vi "get scan info.vi"(5 "piezo z value":i16, 6 "tracking?":bool, 7 "counting photons?":bool, 8 "kalman to host":cluster{"kalman state":T1, "kalman update":bool}, 9 "current location":T3, 10 "scan specification":T2={"z resolution (pixels)"=1000, "iterations per pixel"=28, "iterations per z-scan (=zres*iterperpixel)"=50, "x resolution (pixels)"=100, "y resolution (pixels)"=80, "number of z-lines per volume"=30, "number of repetitions (volumes)"=5, "Pockels cell voltage (bits)"=-1, "Vx center (bits)"=0, "Vy center (bits)"=0, "Vx amplitude (bits)"=40, "Vy amplitude (bits)"=0, "lines to delay between scan start and output"=1, "LSB has acquire control"=FALSE, "Pockels cell bleach voltage"=0}, 11 "counter cluster":T5) -> (3 "scan info":T4)   [LabVIEW 2010]
uses:
  counter_cluster_tagResonant.ctl
  scan_command.ctl
  scan_specification_tagResonant.ctl
  FPGA tracking/integrating single axis kalman state.ctl
  scan message.ctl
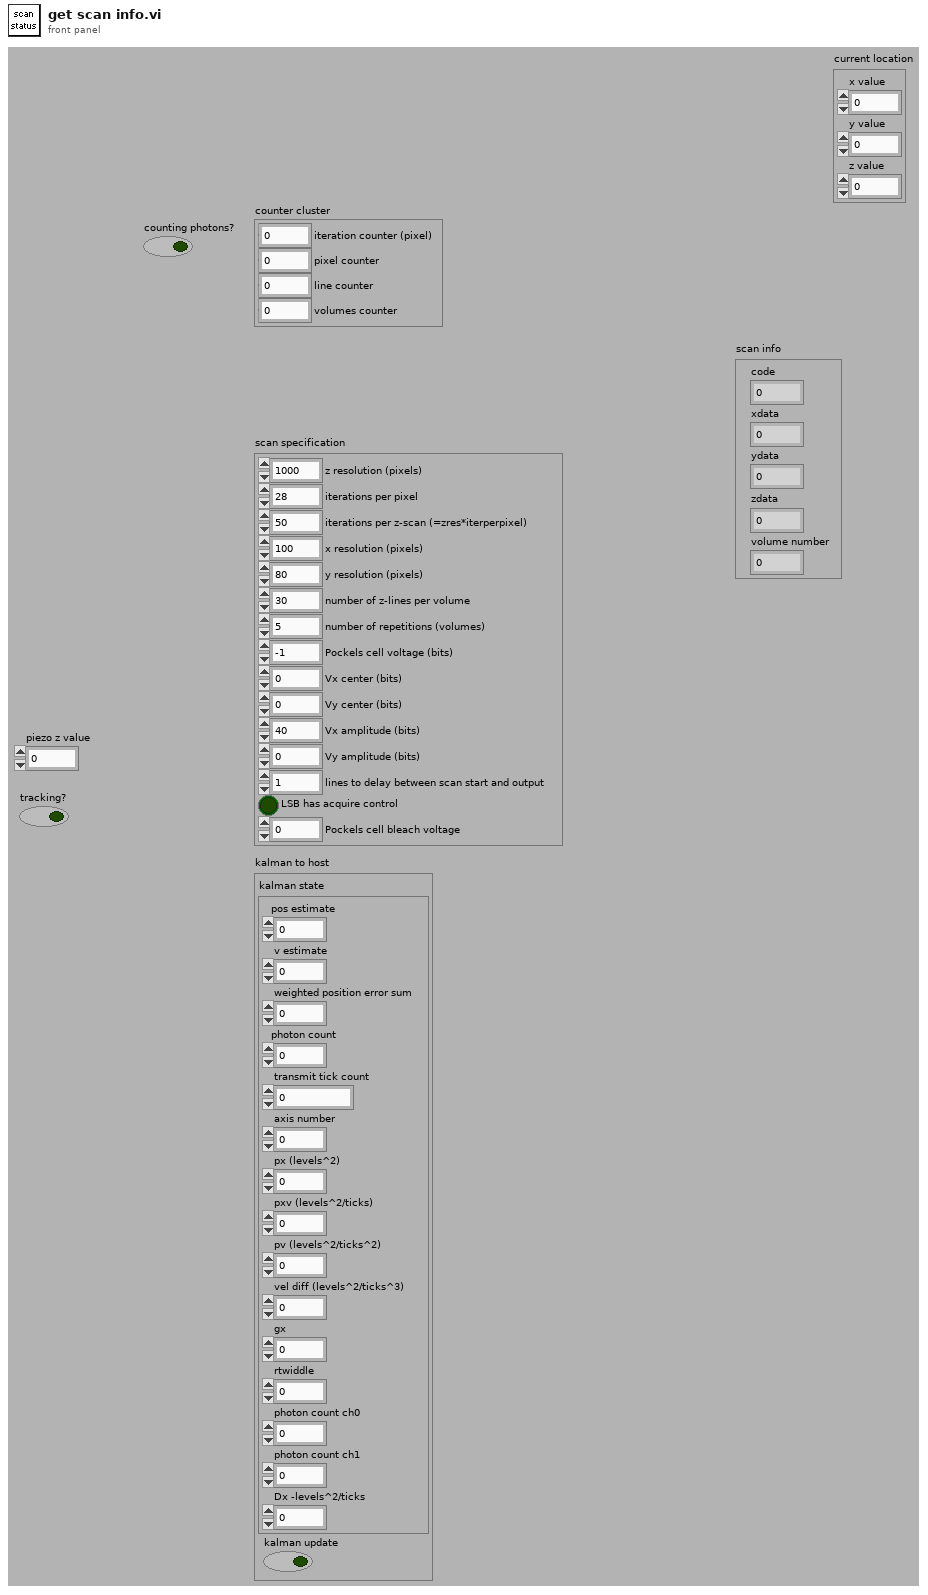
[diagram p1: front panel]
types:
  T1 = typedef "integrating single axis kalman state.ctl" = cluster{"pos estimate":fxp<+/-,32,16>, "v estimate":fxp<+/-,16,0>, "weighted position error sum":fxp<+/-,32,32>, "photon count":u32, "transmit tick count":u32, "axis number":u8, "px (levels^2)":fxp<+,32,19>, "pxv (levels^2/ticks)":fxp<+,32,2>, "pv (levels^2/ticks^2)":fxp<+,32,-14>, "vel diff (levels^2/ticks^3)":fxp<+,24,-22>, "gx":fxp<+,16,8>, "rtwiddle":fxp<+,16,26>, "photon count ch0":u32, "photon count ch1":u32, "Dx -levels^2/ticks":fxp<+,32,19>}
  T2 = typedef "scan_specification_tagResonant.ctl" = cluster{"z resolution (pixels)":u16, "iterations per pixel":u16, "iterations per z-scan (=zres*iterperpixel)":u16, "x resolution (pixels)":u16, "y resolution (pixels)":u16, "number of z-lines per volume":u16, "number of repetitions (volumes)":i32, "Pockels cell voltage (bits)":i16, "Vx center (bits)":i16, "Vy center (bits)":i16, "Vx amplitude (bits)":i16, "Vy amplitude (bits)":i16, "lines to delay between scan start and output":u16, "LSB has acquire control":bool, "Pockels cell bleach voltage":i16}
  T3 = cluster{"x value":i16, "y value":i16, "z value":i16}
  T4 = typedef "scan_command.ctl" = cluster{"code":i32, "xdata":i32, "ydata":i32, "zdata":i32, "volume number":i32}
  T5 = typedef "counter_cluster_tagResonant.ctl" = cluster{"iteration counter (pixel)":u16, "pixel counter":u16, "line counter":i16, "volumes counter":u16}
  T6 = typedef "scan message.ctl" = enum8{"NONE", "VOLUME START", "LINE START", "LINE START TRACKING", "XKALMAN", "YKALMAN", "ZKALMAN"}
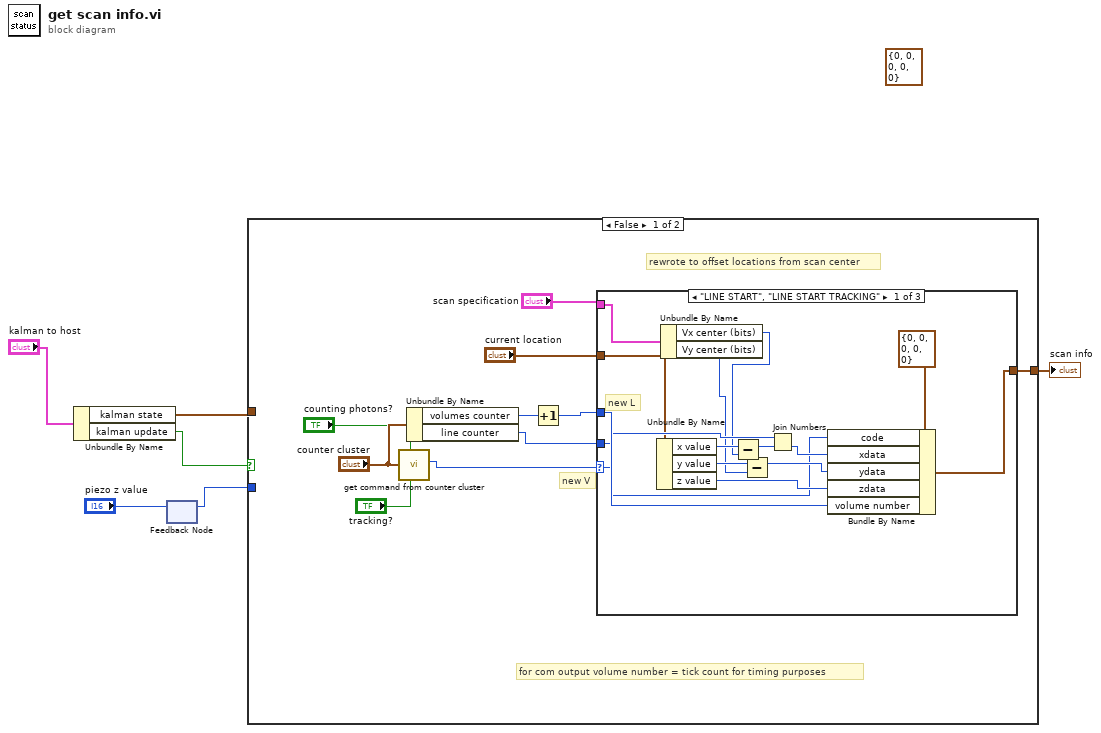
[diagram p0: block diagram]
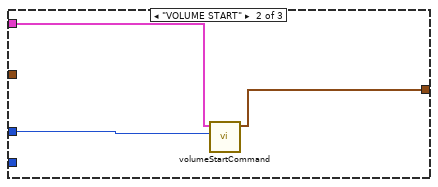
[diagram p2: hidden frame]
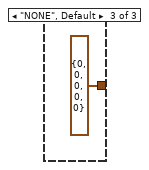
[diagram p3: hidden frame]
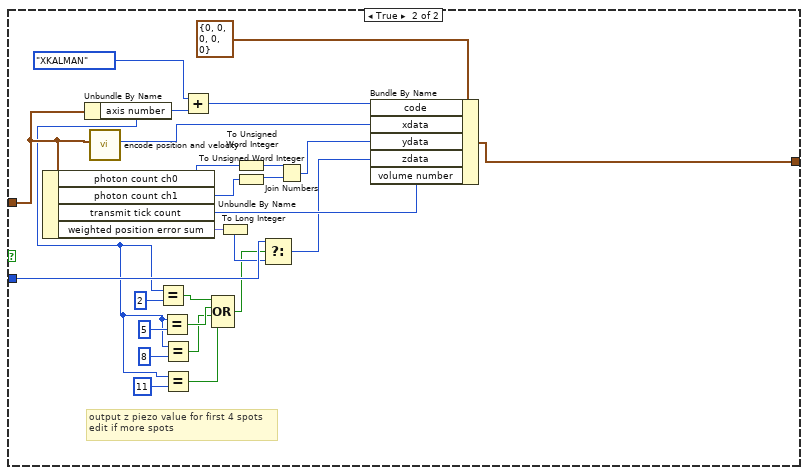
[diagram p4: hidden frame]
diagram:
  (unwired) T4 {"code"=0, "xdata"=0, "ydata"=0, "zdata"=0, "volume number"=0} ("scan info")
  n1 = Unbundle By Name("kalman to host") -> ("kalman state"=w4:T1, "kalman update"=w3:bool)
  n2 = feedback #1() -> (w1:i16)  [unwired: 1 in]
  n3 = feedback-in #1("piezo z value") -> ()
  n4 = case shown="False" w3 {
    tunnel: [w16 w55] -> w6
    tunnel: w4 -> [_ w57]
    tunnel: w1 -> [_ w49]
    frame False {
      # "rewrote to offset locations from scan center"
      # "for com output volume number = tick count for timing purposes"
      # "new V"
      n5 = call "get command from counter cluster.vi"("tracking?"="tracking?", "counting photons?"="counting photons?", "counter cluster"="counter cluster") -> ("command"=w14:T6)  [unwired: 8 in]
      n6 = Unbundle By Name("counter cluster") -> ("volumes counter"=w12:u16, "line counter"=w10:i16)
      n7 = Increment(x=w12) -> (x+1=w11:u16)
      n8 = case shown="\"LINE START\", \"LINE START TRACKING\"" w14 {
        selector: w14 -> [w17 _ _]
        tunnel: w11 -> [w31 w34 _]
        tunnel: [w30 w33 T4 {"code"=0, "xdata"=0, "ydata"=0, "zdata"=0, "volume number"=0} ("scan info")] -> w16
        tunnel: "scan specification" -> [w24 w32 _]
        tunnel: w10 -> [w26 _ _]
        tunnel: "current location" -> [w25 _ _]
        frame "LINE START", "LINE START TRACKING" {
          # "new L"
          n9 = Unbundle By Name(w25) -> ("x value"=w22:i16, "y value"=w20:i16, "z value"=w28:i16)
          n10 = Unbundle By Name(w24) -> ("Vx center (bits)"=w19:i16, "Vy center (bits)"=w18:i16)
          n11 = Subtract(x=w22, y=w19) -> (x-y=w23:i16)
          n12 = Subtract(x=w20, y=w18) -> (x-y=w21:i16)
          n13 = Join Numbers(hi=w26, lo=w23) -> ((hi.lo)=w27:u32)
          n14 = Bundle By Name(cluster=T4 {"code"=0, "xdata"=0, "ydata"=0, "zdata"=0, "volume number"=0} ("scan info"), "code"=w17, "xdata"=w27, "ydata"=w21, "zdata"=w28, "volume number"=w31) -> (w30:T4)
        }
        frame "VOLUME START" {
          n15 = call "volumeStartCommand.vi"("volume number"=w34, "scan specification"=w32) -> ("scan info"=w33:T4)  [unwired: 9 in]
        }
        frame "NONE", Default {
        }
      }
    }
    frame True {
      # "output z piezo value for first 4 spots\nedit if more spots"
      n16 = Unbundle By Name(w57) -> ("photon count ch0"=w54:u32, "photon count ch1"=w53:u32, "transmit tick count"=w56:u32, "weighted position error sum"=w47:fxp<+/-,32,32>)
      n17 = Unbundle By Name(w57) -> ("axis number"=w36:u8)
      n18 = call "encode position and velocity.vi"("state"=w57) -> ("pos and vel"=w58:u32)  [unwired: 10 in]
      n19 = Equal?(x=w36, y=u8 2) -> (x = y?=w40:bool)
      n20 = Equal?(x=w36, y=u8 5) -> (x = y?=w39:bool)
      n21 = Equal?(x=w36, y=u8 8) -> (x = y?=w38:bool)
      n22 = Equal?(x=w36, y=u8 11) -> (x = y?=w37:bool)
      n23 = Add(x=scan_message."XKALMAN" ("command"), y=w36) -> (x+y=w59:u8)
      n24 = Compound Arithmetic op=OR(w40, w39, w38, w37) -> (w41:bool)
      n25 = To Long Integer(number=w47) -> (32bit integer=w46:i32)
      n26 = To Unsigned Word Integer(number=w54) -> (unsigned 16bit integer=w52:u16)
      n27 = To Unsigned Word Integer(number=w53) -> (unsigned 16bit integer=w51:u16)
      n28 = Select(t=w49, s=w41, f=w46) -> (s? t:f=w45:i32)
      n29 = Join Numbers(hi=w52, lo=w51) -> ((hi.lo)=w50:u32)
      n30 = Bundle By Name(cluster=T4 {"code"=0, "xdata"=0, "ydata"=0, "zdata"=0, "volume number"=0} ("scan info"), "code"=w59, "xdata"=w58, "ydata"=w50, "zdata"=w45, "volume number"=w56) -> (w55:T4)
    }
  }
  "scan info" <- w6
